vi "Set Exp sel #.vi"(8 "error in (no error)":errorcluster, 10 "Exp sel #":i32, 11 "Experiments_group in":refnum<class "Experiments_group.lvclass">) -> (0 "error out":errorcluster, 3 "Experiments_group out":refnum<class "Experiments_group.lvclass">)   [LabVIEW 2019, in "Experiments_group.lvclass"]
uses:
  Experiments_group.lvclass
  Experiments_group.lvclass/Experiments_group.ctl
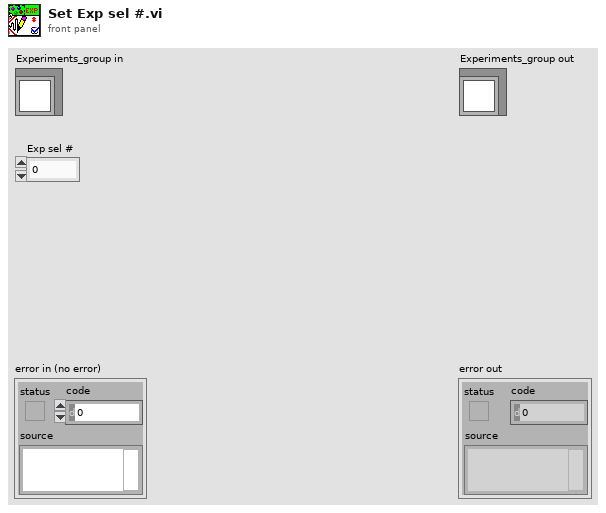
[diagram p1: front panel]
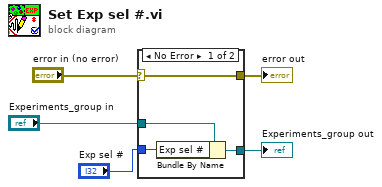
[diagram p0: block diagram]
diagram:
  n1 = case shown="No Error" "error in (no error)" {
    selector: "error in (no error)" -> [w9 w10]
    tunnel: [w9 w10] -> w4
    tunnel: [w7 w11] -> w2
    tunnel: "Experiments_group in" -> [w8 w11]
    tunnel: "Exp sel #" -> [w6 _]
    frame No Error {
      n2 = Bundle By Name(cluster=w8, "Exp sel #"=w6) -> (w7:refnum<class "Experiments_group.lvclass">)
    }
    frame Error {
    }
  }
  "error out" <- w4
  "Experiments_group out" <- w2
